vi "IVC_OC200_Global.vi"() -> ()   [LabVIEW 2019]
panel:
  out "IVC_OC200_ST":u32(colorbox)
  out "IVC_OC200_P2":dbl
  out "IVC_OC200_P1":dbl
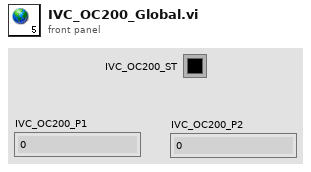
[diagram p1: front panel]
diagram:
